vi "mcc_usb202_close.vi"(6 "error in":errorcluster, 11 "task in":refnum<k24>) -> (0 "status":bool=TRUE, 4 "error out":errorcluster={"status"=TRUE, "code"=0, "source"=""})   [LabVIEW 2019]
uses:
  C:/Program Files/National Instruments/LabVIEW 2019/vi.lib/ULx/ULx_LV.dll
  Program Files/National Instruments/LabVIEW 2019/vi.lib/ULx/ULx_LV.dll
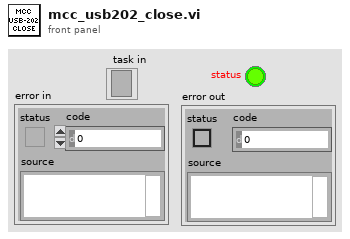
[diagram p1: front panel]
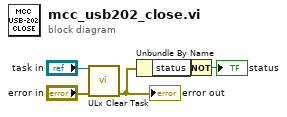
[diagram p0: block diagram]
diagram:
  n1 = call <vilib>:"ULx Clear Task.vi"("task in"="task in", "error in"="error in") -> ("error out"=w3:errorcluster)  [unwired: 13 in]
  "error out" <- w3
  n2 = Unbundle By Name(w3) -> ("status"=w2:bool)
  n3 = Not(x=w2) -> (.not. x?=→"status":bool)
